vi "ExFileReadNDisplayTifCalNI.vi"() -> ()   [LabVIEW 2010]
panel:
  out "XY Graph":cluster{"Array":dbl[], "Array F32":sgl[]}(graph)
  in  "Full File Name":path=path "C:/Program Files/SIToolKit/LabVIEW/Data Files/CALIBHGARGON.TIF"
  in  "?":bool
  in  "FileType":u32=67174400
  out "error out":errorcluster
  in  "error in (no error)":errorcluster
  # "ExReadFileNDisplayTifCalNI.vi\nThis example will read in a file of the selected data type and display all frames. When finished viewing data, make sure to use the STOP button to close the display.\nIf there is a calibration in the file (TIF) then it will update the x axis\nfor that calibration"
  # "File Types:\nSPE = 67371008\nTIF   = 67174400\nPMI  = 67436544"
  # "Browse match pattern is set to *.spe.  Modify this if different file type is needed."
  # "This will properly close\nthe image and\ndeallocate memory."
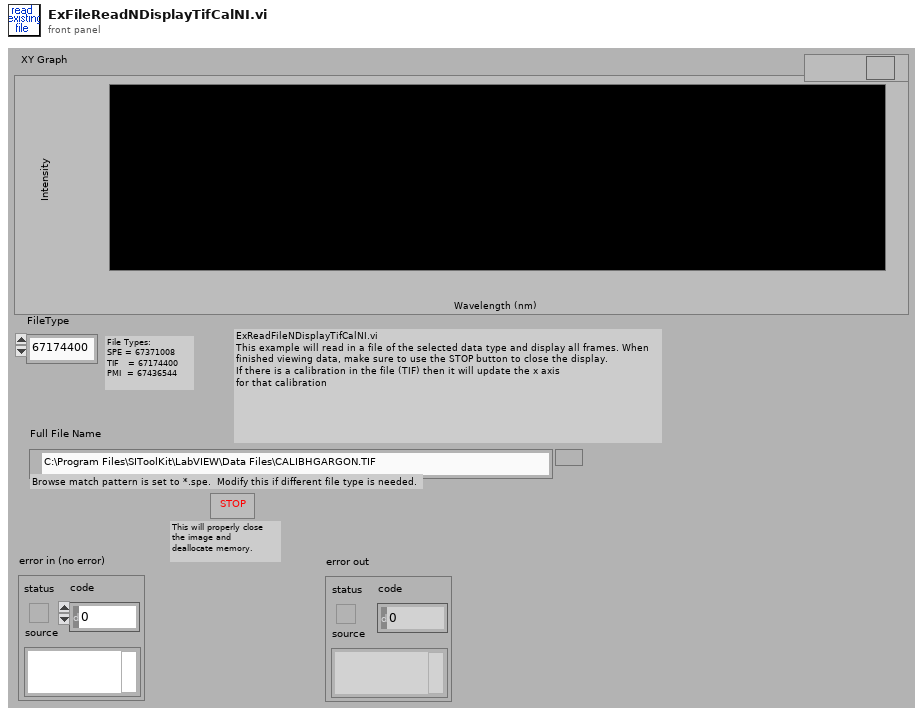
[diagram p1: front panel]
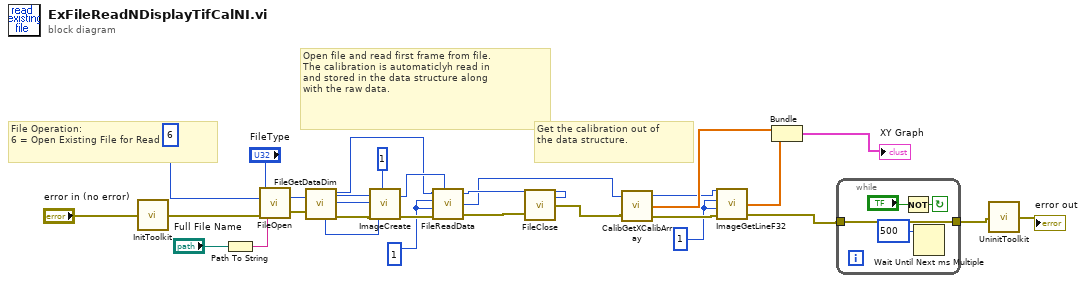
[diagram p0: block diagram]
diagram:
  w3 = 1
  w15 = 1
  # "Get the calibration out of\nthe data structure."
  # "Open file and read first frame from file.\nThe calibration is automaticlyh read in\nand stored in the data structure along\nwith the raw data."
  # "File Operation:\n6 = Open Existing File for Read"
  n1 = call <userlib>:"InitToolkit.vi"("error in"="error in (no error)") -> ("error out"=w28:errorcluster)
  n2 = Path To String(path="Full File Name") -> (string=w17:string)
  n3 = call <userlib>:"FileOpen.vi"("error in"=w28, "File Operations"=u32 6 ("File Operation"), "FileName"=w17, "File Type"="FileType") -> ("error out"=w26:errorcluster, "File Handle"=w25:u32)
  n4 = call <userlib>:"FileGetDataDim.vi"("File Handle"=w25, "error in"=w26) -> ("Data Type"=w21:u32, "File Handle"=w13:u32, "X dim"=w23:u32, "Y dim"=w22:u32, "error out"=w24:errorcluster)  [unwired: 1 out]
  n5 = call <userlib>:"ImageCreate.vi"("X dimension"=w23, "Y dimension"=w22, "Data Type"=w21, "error in"=w24, "Number Of Frames"=1) -> ("Image Handle"=w14:u32, "error out"=w16:errorcluster)
  n6 = call <userlib>:"FileReadData.vi"("File Handle"=w13, "Start Frame"=w15, "End Frame"=w15, "error in"=w16, "Image Handle"=w14) -> ("File Handle"=w12:u32, "Image Handle"=w10:u32, "error out"=w11:errorcluster)
  n7 = call <userlib>:"FileClose.vi"("error in"=w11, "File Handle"=w12) -> ("error out"=w7:errorcluster)
  n8 = call <userlib>:"CalibGetXCalibArray.vi"("Data Handle"=w10, "error in (no error)"=w7) -> ("Data Handle"=w2:u32, "Array"=w8:dbl[], "error out"=w6:errorcluster)
  n9 = call <userlib>:"ImageGetLineF32.vi"("error in"=w6, "Z Position"=w3, "Y Position"=w3, "Data Handle"=w2) -> ("error out"=w5:errorcluster, "Array F32"=w9:sgl[])  [unwired: 1 out]
  n10 = Bundle("Array"=w8, "Array F32"=w9) -> (→"XY Graph":cluster{"Array":dbl[], "Array F32":sgl[]})  [unwired: 1 in]
  n11 = while {
    tunnel: w5 -> [w31]
    tunnel: [w31] -> w4
    stop <- w33 continue-if-true
    n12 = Not(x="?") -> (.not. x?=w33:bool)
    n13 = Wait Until Next ms Multiple(millisecond multiple=500) -> ()  [unwired: 1 out]
  }
  n14 = call <userlib>:"UninitToolkit.vi"("error in"=w4) -> ("error out"=→"error out":errorcluster)
